vi "Mouvement encodeur.vi"(6 "Vitesse initiale":dbl, 7 "Temps acceleration":dbl, 8 "Reverse":bool, 9 "Left":bool, 10 "Right":bool, 11 "Distance":dbl) -> ()   [LabVIEW 2016]
uses:
  <vilib>/Rock Robotics/WPI/Utilities/WPI_GetSetVariantRefNum.vi
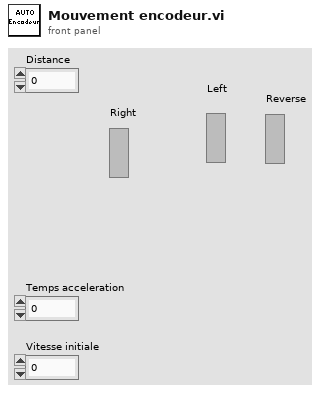
[diagram p1: front panel]
types:
  T1 = typedef "WPI_EncoderDevRef.ctl" = cluster{"DevStatus":errorcluster, "EncoderIndex":T2, "CounterIndex":T3, "DistancePerCount":dbl, "Decoding Type":T4}
  T2 = typedef "FPGA_EncoderIdx.ctl" = enum8{"Enc 0", "Enc 1", "Enc 2", "Enc 3", "Enc 4", "Enc 5", "Enc 6", "Enc 7", "Invalid"}
  T3 = typedef "FPGA_CounterCtrSystemIndex.ctl" = enum8{"Ctr 0", "Ctr 1", "Ctr 2", "Ctr 3", "Ctr 4", "Ctr 5", "Ctr 6", "Ctr 7", "Invalid"}
  T4 = typedef "WPI_EncoderType.ctl" = enum16{"1x", "2x", "4x"}
  T5 = typedef "WPI_RobotDriveDevRef.ctl" = cluster{"DevStatus":errorcluster, "Motors[]":T6[], "Square Inputs":bool, "Max Output":dbl}
  T6 = typedef "WPI_MotorControlDeviceRef.ctl" = cluster{"DeviceStatus":errorcluster, "Type":T7, "PWM":cluster{"PWM Channel":T8, "DeadBand":T9}, "CAN":cluster{"Device Number":u8, "SetOutput VI Ref":variant, "GetOutput VI Ref":variant, "Enable VI Ref":variant, "Disable VI Ref":variant, "Data":variant}, "Invert":bool}
  T7 = typedef "WPI_MotorControlType.ctl" = enum16{"PWM", "CAN"}
  T8 = typedef "FPGA_DIOPWMChannel.ctl" = enum8{"PWM 0", "PWM 1", "PWM 2", "PWM 3", "PWM 4", "PWM 5", "PWM 6", "PWM 7", "PWM 8", "PWM 9", "PWM MXP 0", "PWM MXP 1", "PWM MXP 2", "PWM MXP 3", "PWM MXP 4", "PWM MXP 5", "PWM MXP 6", "PWM MXP 7", "PWM MXP 8", "PWM MXP 9", "Invalid"}
  T9 = typedef "WPI_PWMDeadband.ctl" = cluster{"Name":string, "maxPositivePwm":i32, "minPositivePwm":i32, "centerPwm":i32, "maxNegativePwm":i32, "minNegativePwm":i32, "angularRange":u16}
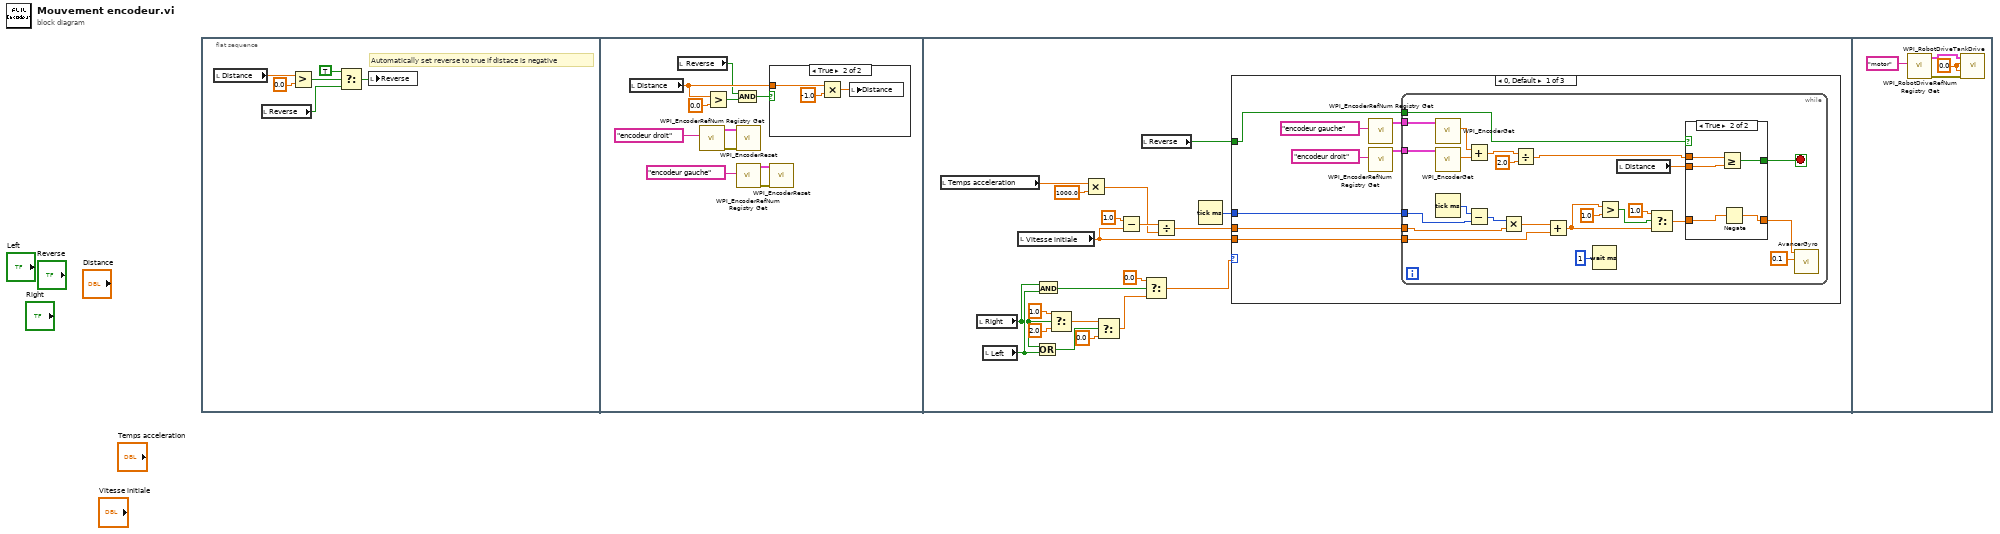
[diagram p0: block diagram]
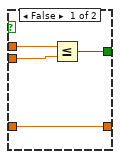
[diagram p3: hidden frame]
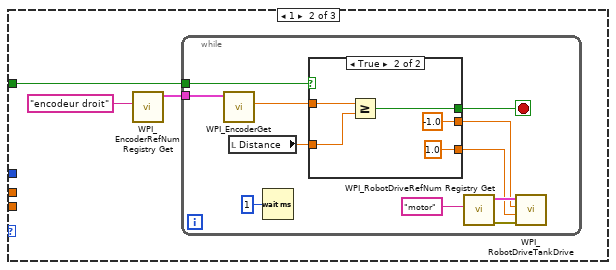
[diagram p4: hidden frame]
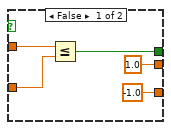
[diagram p5: hidden frame]
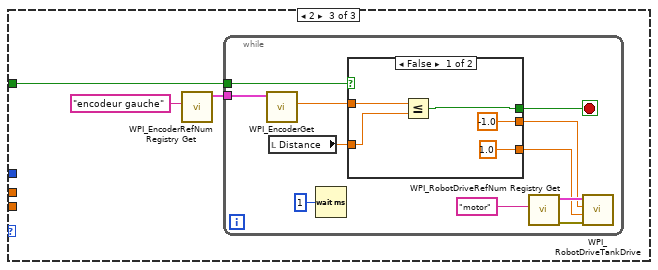
[diagram p6: hidden frame]
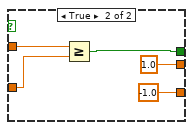
[diagram p7: hidden frame]
diagram:
  n1 = flat-sequence {
    frame #0 {
      # "Automatically set reverse to true if distace is negative"
      n2 = local read "Distance"() -> (w5:dbl)
      n3 = local read "Reverse"() -> (w3:bool)
      n4 = Greater?(x=w5, y=0.0) -> (0:w4:bool)
      n5 = Select(t=TRUE, s=w4, f=w3) -> (s? t:f=w1:bool)
      n6 = local write "Reverse"(w1) -> ()
    }
    frame #1 {
      n7 = local read "Distance"() -> (w11:dbl)
      n8 = local read "Reverse"() -> (w7:bool)
      n9 = call <vilib>:"WPI_EncoderRefNum Registry Get.vi"("refnum name"="encodeur droit") -> ("error out"=w12:errorcluster, "EncoderDevRef"=w13:T1)  [unwired: 9 in]
      n10 = Greater?(x=w11, y=0.0) -> (0:w9:bool)
      n11 = And(x=w7, y=w9) -> (x .and. y?=w10:bool)
      n12 = call <vilib>:"WPI_EncoderReset.vi"("error in (no error)"=w12, "EncoderDevRef"=w13) -> ()  [unwired: 8 in, 2 out]
      n13 = call <vilib>:"WPI_EncoderRefNum Registry Get.vi"("refnum name"="encodeur gauche") -> ("error out"=w14:errorcluster, "EncoderDevRef"=w15:T1)  [unwired: 9 in]
      n14 = case shown="True" w10 {
        tunnel: w11 -> [_ w20]
        frame False {
        }
        frame True {
          n15 = Multiply(x=w20, y=-1.0) -> (x*y=w18:dbl)
          n16 = local write "Distance"(w18) -> ()
        }
      }
      n17 = call <vilib>:"WPI_EncoderReset.vi"("error in (no error)"=w14, "EncoderDevRef"=w15) -> ()  [unwired: 8 in, 2 out]
    }
    frame #2 {
      n18 = local read "Temps acceleration"() -> (w28:dbl)
      n19 = local read "Right"() -> (w32:bool)
      n20 = local read "Left"() -> (w33:bool)
      n21 = local read "Vitesse initiale"() -> (w21:dbl)
      n22 = Or(x=w32, y=w33) -> (x .or. y?=w34:bool)
      n23 = And(x=w32, y=w33) -> (x .and. y?=w31:bool)
      n24 = Select(t=1.0, s=w32, f=2.0) -> (s? t:f=w38:dbl)
      n25 = Multiply(x=w28, y=1000.0) -> (x*y=w24:dbl)
      n26 = Select(t=w38, s=w34, f=0.0) -> (s? t:f=w35:dbl)
      n27 = Subtract(x=1.0, y=w21) -> (x-y=w25:dbl)
      n28 = local read "Reverse"() -> (w29:bool)
      n29 = Select(t=0.0, s=w31, f=w35) -> (s? t:f=w36:dbl)
      n30 = Divide(x=w25, y=w24) -> (x/y=w22:dbl)
      n31 = Tick Count (ms)() -> (millisecond timer value=w23:u32)
      n32 = case shown="0, Default" w36 {
        tunnel: w29 -> [w44 w82 w106]
        tunnel: w23 -> [w43 _ _]
        tunnel: w22 -> [w42 _ _]
        tunnel: w21 -> [w41 _ _]
        frame 0, Default {
          n33 = call <vilib>:"WPI_EncoderRefNum Registry Get.vi"("refnum name"="encodeur gauche") -> ("EncoderDevRef"=w48:T1)  [unwired: 9 in, 1 out]
          n34 = call <vilib>:"WPI_EncoderRefNum Registry Get.vi"("refnum name"="encodeur droit") -> ("EncoderDevRef"=w47:T1)  [unwired: 9 in, 1 out]
          n35 = while {
            tunnel: w47 -> [w72]
            tunnel: w48 -> [w71]
            tunnel: w44 -> [w63]
            tunnel: w43 -> [w61]
            tunnel: w42 -> [w58]
            tunnel: w41 -> [w56]
            stop <- w65 stop-if-true
            n36 = call <vilib>:"WPI_EncoderGet.vi"("EncoderDevRef"=w71) -> ("Distance"=w70:dbl)  [unwired: 5 in, 5 out]
            n37 = call <vilib>:"WPI_EncoderGet.vi"("EncoderDevRef"=w72) -> ("Distance"=w69:dbl)  [unwired: 5 in, 5 out]
            n38 = Tick Count (ms)() -> (millisecond timer value=w60:u32)
            n39 = Add(x=w70, y=w69) -> (x+y=w68:dbl)
            n40 = Subtract(x=w60, y=w61) -> (x-y=w59:u32)
            n41 = Multiply(x=w59, y=w58) -> (x*y=w57:dbl)
            n42 = Divide(x=w68, y=2.0) -> (x/y=w66:dbl)
            n43 = Add(x=w57, y=w56) -> (x+y=w53:dbl)
            n44 = Wait (ms)(milliseconds to wait=u32 1) -> ()  [unwired: 1 out]
            n45 = Greater?(x=w53, y=1.0) -> (0:w54:bool)
            n46 = local read "Distance"() -> (w64:dbl)
            n47 = Select(t=1.0, s=w54, f=w53) -> (s? t:f=w52:dbl)
            n48 = case shown="True" w63 {
              tunnel: w66 -> [w76 w81]
              tunnel: [w74 w80] -> w65
              tunnel: w64 -> [w75 w79]
              tunnel: [w73 w78] -> w50
              tunnel: w52 -> [w73 w77]
              frame False {
                n49 = Less Or Equal?(x=w76, y=w75) -> (x <= y?=w74:bool)
              }
              frame True {
                n50 = Greater Or Equal?(x=w81, y=w79) -> (x >= y?=w80:bool)
                n51 = Negate(x=w77) -> (-x=w78:dbl)
              }
            }
            n52 = call "AvancerGyro.vi"("Ajustement"=0.1, "Vitesse"=w50) -> ()  [unwired: 10 in]
          }
        }
        frame 1 {
          n53 = call <vilib>:"WPI_EncoderRefNum Registry Get.vi"("refnum name"="encodeur droit") -> ("EncoderDevRef"=w83:T1)  [unwired: 9 in, 1 out]
          n54 = while {
            tunnel: w83 -> [w95]
            tunnel: w82 -> [w88]
            stop <- w94 stop-if-true
            n55 = call <vilib>:"WPI_EncoderGet.vi"("EncoderDevRef"=w95) -> ("Distance"=w93:dbl)  [unwired: 5 in, 5 out]
            n56 = local read "Distance"() -> (w92:dbl)
            n57 = Wait (ms)(milliseconds to wait=u32 1) -> ()  [unwired: 1 out]
            n58 = case shown="True" w88 {
              tunnel: [w98 w105] -> w94
              tunnel: w93 -> [w100 w104]
              tunnel: w92 -> [w99 w103]
              tunnel: [-1.0 ("Right axis value") 1.0 ("Right axis value")] -> w87
              tunnel: [1.0 ("Left axis value") -1.0 ("Left axis value")] -> w86
              frame False {
                n59 = Less Or Equal?(x=w100, y=w99) -> (x <= y?=w98:bool)
              }
              frame True {
                n60 = Greater Or Equal?(x=w104, y=w103) -> (x >= y?=w105:bool)
              }
            }
            n61 = call <vilib>:"WPI_RobotDriveRefNum Registry Get.vi"("refnum name"="motor") -> ("error out"=w91:errorcluster, "RobotDriveDevRef"=w90:T5)  [unwired: 9 in]
            n62 = call <vilib>:"WPI_RobotDriveTankDrive.vi"("error in (no error)"=w91, "Right axis value"=w87, "Left axis value"=w86, "RobotDriveDevRef"=w90) -> ()  [unwired: 5 in, 3 out]
          }
        }
        frame 2 {
          n63 = call <vilib>:"WPI_EncoderRefNum Registry Get.vi"("refnum name"="encodeur gauche") -> ("EncoderDevRef"=w108:T1)  [unwired: 9 in, 1 out]
          n64 = while {
            tunnel: w108 -> [w119]
            tunnel: w106 -> [w112]
            stop <- w118 stop-if-true
            n65 = call <vilib>:"WPI_EncoderGet.vi"("EncoderDevRef"=w119) -> ("Distance"=w117:dbl)  [unwired: 5 in, 5 out]
            n66 = local read "Distance"() -> (w116:dbl)
            n67 = Wait (ms)(milliseconds to wait=u32 1) -> ()  [unwired: 1 out]
            n68 = case shown="False" w112 {
              tunnel: [w122 w129] -> w118
              tunnel: w117 -> [w124 w128]
              tunnel: w116 -> [w123 w127]
              tunnel: [-1.0 ("Left axis value") 1.0 ("Left axis value")] -> w111
              tunnel: [1.0 ("Right axis value") -1.0 ("Right axis value")] -> w110
              frame False {
                n69 = Less Or Equal?(x=w124, y=w123) -> (x <= y?=w122:bool)
              }
              frame True {
                n70 = Greater Or Equal?(x=w128, y=w127) -> (x >= y?=w129:bool)
              }
            }
            n71 = call <vilib>:"WPI_RobotDriveRefNum Registry Get.vi"("refnum name"="motor") -> ("error out"=w113:errorcluster, "RobotDriveDevRef"=w114:T5)  [unwired: 9 in]
            n72 = call <vilib>:"WPI_RobotDriveTankDrive.vi"("error in (no error)"=w113, "Right axis value"=w110, "Left axis value"=w111, "RobotDriveDevRef"=w114) -> ()  [unwired: 5 in, 3 out]
          }
        }
      }
    }
    frame #3 {
      w133 = 0.0 ("Left axis value")
      n73 = call <vilib>:"WPI_RobotDriveRefNum Registry Get.vi"("refnum name"="motor") -> ("error out"=w130:errorcluster, "RobotDriveDevRef"=w131:T5)  [unwired: 9 in]
      n74 = call <vilib>:"WPI_RobotDriveTankDrive.vi"("error in (no error)"=w130, "Right axis value"=w133, "Left axis value"=w133, "RobotDriveDevRef"=w131) -> ()  [unwired: 5 in, 3 out]
    }
  }
